vi "CreateFileEvents.vi"(11 "Date/time":string) -> (0 "error out":errorcluster, 3 "Byte Stream File out":refnum<file>)   [LabVIEW 2018]
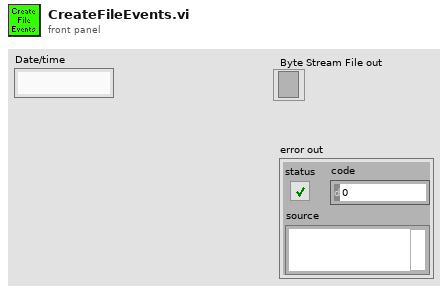
[diagram p1: front panel]
types:
  T1 = typedef "NetComm_MatchType.ctl" = enum32{"None", "Practice", "Qualification", "Elimination"}
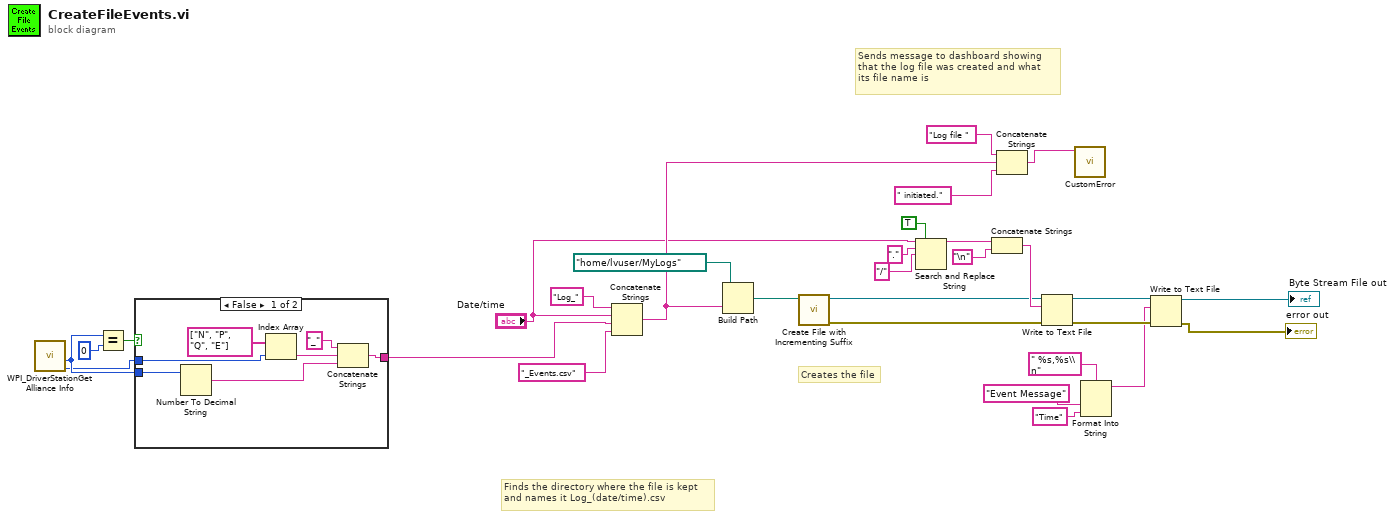
[diagram p0: block diagram]
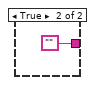
[diagram p2: hidden frame]
diagram:
  # "Finds the directory where the file is kept\nand names it Log_(date/time).csv"
  # "Creates the file"
  # "Sends message to dashboard showing\nthat the log file was created and what \nits file name is"
  n1 = call <vilib>:"WPI_DriverStationGet Alliance Info.vi"() -> ("Match Type"=w18:T1, "Match Number"=w24:u16)  [unwired: 6 in, 4 out]
  n2 = Equal?(x=w24, y=u16 0) -> (x = y?=w26:bool)
  n3 = case shown="False" w26 {
    tunnel: [w36 ""] -> w19
    tunnel: w24 -> [w37 _]
    tunnel: w18 -> [w33 _]
    frame False {
      n4 = Number To Decimal String(number=w37) -> (decimal integer string=w31:string)  [unwired: 1 in]
      n5 = Index Array(array=string[] ["N", "P", "Q", "E"], index=w33) -> (element=w32:string)
      n6 = Concatenate Strings("_" ("string"), w32, w31) -> (w36:string)
    }
    frame True {
    }
  }
  n7 = Concatenate Strings("Log_" ("string"), "Date/time", w19, "_Events.csv" ("string")) -> (w20:string)
  n8 = Build Path(base path=path "/home/lvuser/MyLogs", name or relative path=w20) -> (appended path=w21:path)
  n9 = call <vilib>:"Create File with Incrementing Suffix.vi"("file path"=w21) -> ("error out"=w11:errorcluster, "refnum out"=w10:refnum<file>)  [unwired: 8 in, 1 out]
  n10 = Search and Replace String(replace all?=TRUE ("replace all? (F)"), input string="Date/time", search string=".", replace string="/" ("search string")) -> (result string=w13:string)  [unwired: 4 in, 3 out]
  n11 = Concatenate Strings(w13, "\n") -> (w16:string)
  n12 = Concatenate Strings("Log file " ("Source"), w20, " initiated." ("string")) -> (w28:string)
  n13 = Write to Text File(file (use dialog)=w10, text=w16, error in=w11) -> (refnum out=w8:refnum<file>, error out=w7:errorcluster)  [unwired: 1 in, 1 out]
  n14 = call "CustomError.vi"("String"=w28) -> ()  [unwired: 10 in, 1 out]
  n15 = Format Into String(format string=" %s,%s\\n", "Event Message" ("input 2"), "Time" ("input 2")) -> (resulting string=w3:string)  [unwired: 2 in, 1 out]
  n16 = Write to Text File(file (use dialog)=w8, text=w3, error in=w7) -> (refnum out=→"Byte Stream File out":refnum<file>, error out=→"error out":errorcluster)  [unwired: 1 in, 1 out]
